vi "Open LVM Data.vi"(0 "Filename":path=path "E:/LabVIEW/Data/Test Data/Subj-Austin_Trial-1_Condition-None.lvm", 1 "VI reference":refnum<vi>, 11 "Error In":errorcluster) -> (4 "Filename Out":path=path "E:/LabVIEW/Data/Test Data/Subj-Austin_Trial-1_Condition-None.lvm" caption="Filename", 6 "All Data":dynamicdata(graph), 10 "EGG?":bool, 15 "Error Out":errorcluster)   [LabVIEW 2020]
panel:
  out "Signals (Array)":string[](array[string])
  out "EGG":dynamicdata(graph)
  out "Upper SPL":dbl
  out "Comment":string
  out "Audio":dynamicdata(graph)
  out "SPL":dynamicdata(graph)
  out "Pressure":dynamicdata(graph)
  out "Flow":dynamicdata(graph)
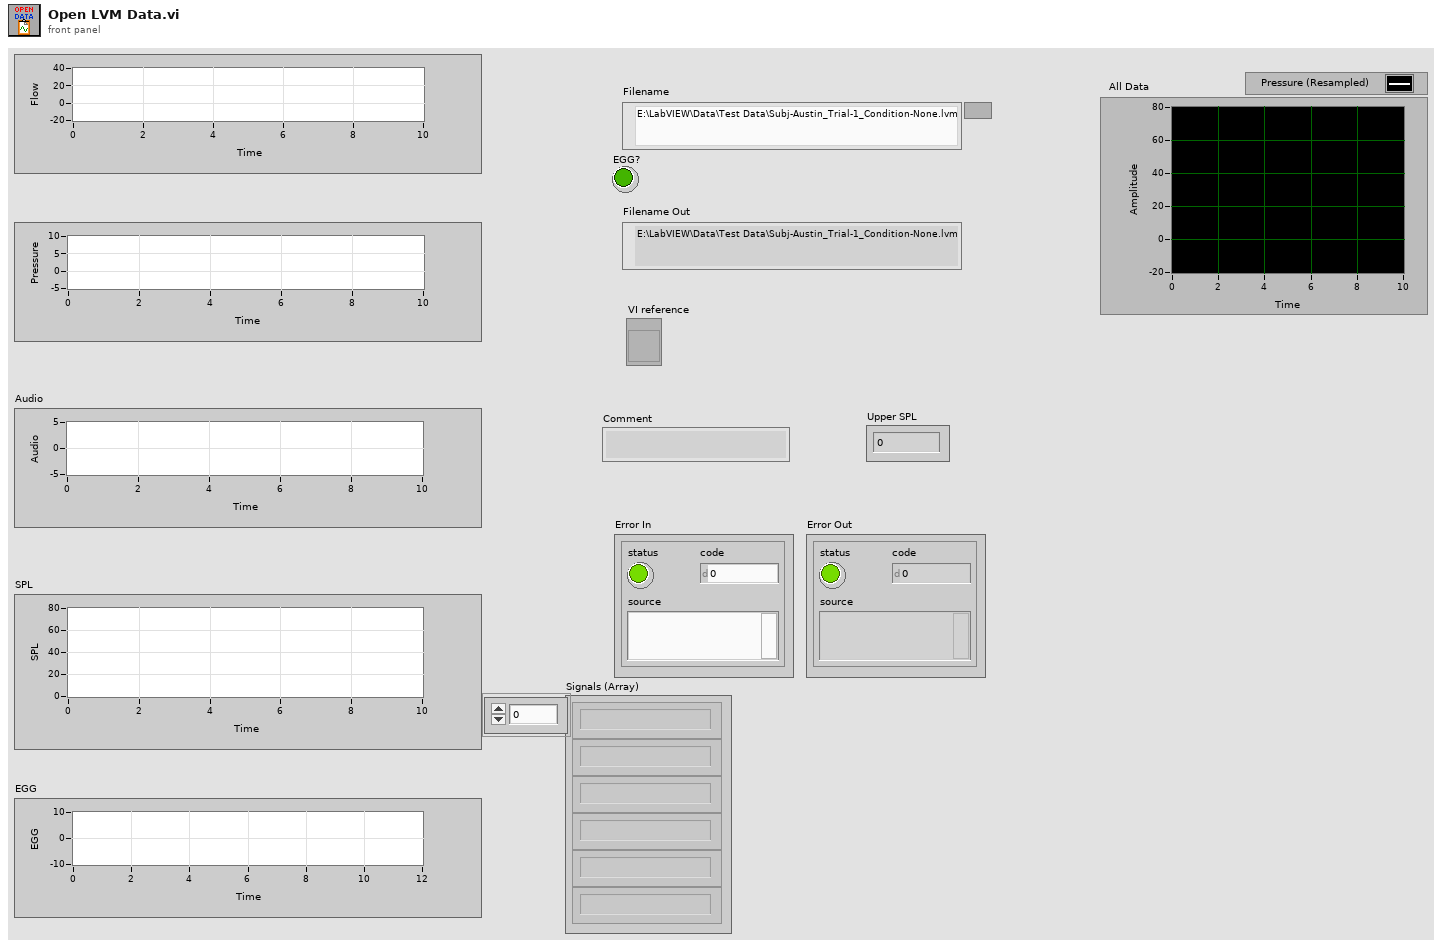
[diagram p1: front panel]
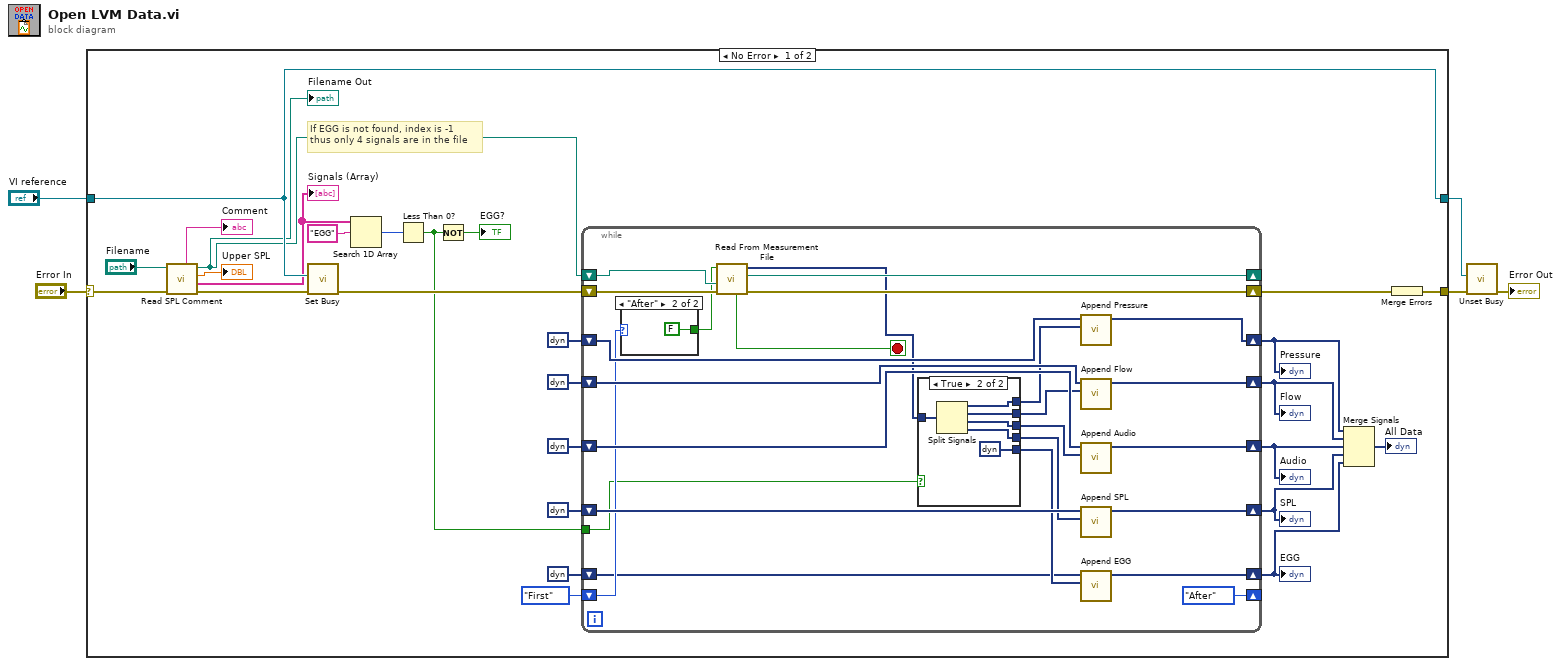
[diagram p0: block diagram]
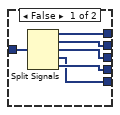
[diagram p2: hidden frame]
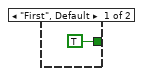
[diagram p3: hidden frame]
diagram:
  n1 = case shown="No Error" "Error In" {
    selector: "Error In" -> [w20 w73]
    tunnel: [w32 w73] -> w4
    tunnel: "VI reference" -> [w25 w72]
    tunnel: [w25 w72] -> w1
    frame No Error {
      # "If EGG is not found, index is -1\nthus only 4 signals are in the file"
      n2 = call "Read SPL Comment.vi"("error in (no error)"=w20, "Filename"="Filename") -> ("error out"=w14:errorcluster, "Signals"=w15:string[], "Upper SPL"=→"Upper SPL":dbl, "Filename Out"=w17:path, "Comment"=→"Comment":string)  [unwired: 5 in]
      "Filename Out" <- w17
      "Signals (Array)" <- w15
      n3 = call <vilib>:"Set Busy.vi"("error in (no error)"=w14, "VI reference (current VI)"=w25) -> ("error out"=w21:errorcluster)  [unwired: 8 in, 1 out]
      n4 = Search 1D Array(1D array=w15, element="EGG") -> (index of element=w22:i32)  [unwired: 1 in]
      n5 = Less Than 0?(x=w22) -> (x < 0?=w13:bool)
      n6 = Not(x=w13) -> (.not. x?=→"EGG?":bool)
      n7 = while {
        shift-right: [w56] -> w27
        shift-left: w21 -> [w55]
        shift-right: [w57] -> _
        shift-left: w17 -> [w54]
        shift-right: [w45] -> w11
        shift-left: dynamicdata [] ("Waveform Graph") -> [w52]
        shift-right: [w41] -> w10
        shift-left: dynamicdata [] ("Waveform Graph") -> [w51]
        shift-right: [w44] -> w9
        shift-left: dynamicdata [] ("Waveform Graph") -> [w50]
        shift-right: [w42] -> w8
        shift-left: dynamicdata [] ("Waveform Graph") -> [w49]
        shift-right: [enum16{"First", "After"}."After"] -> _
        shift-left: enum16{"First", "After"}."First" -> [w40]
        shift-right: [w34] -> w7
        shift-left: dynamicdata [] ("Waveform Graph") -> [w35]
        tunnel: w13 -> [w33]
        stop <- w53 stop-if-true
        n8 = case shown="\"After\"" w40 {
          tunnel: [TRUE ("Reset") FALSE ("Reset")] -> w39
          frame "First", Default {
          }
          frame "After" {
          }
        }
        n9 = call "Read From Measurement File"("error in (no error)"=w55, "Filename"=w54, "Reset"=w39) -> ("error out"=w56:errorcluster, "Filename Out"=w57:path, "Signals"=w43:dynamicdata, "EOF?"=w53:bool)  [unwired: 3 in, 2 out]
        n10 = case shown="True" w33 {
          tunnel: [w63 w67] -> w48
          tunnel: [w62 w66] -> w47
          tunnel: [w61 w65] -> w46
          tunnel: w43 -> [w60 w69]
          tunnel: [w59 w64] -> w37
          tunnel: [w58 dynamicdata [] ("Waveform Graph")] -> w36
          frame False {
            n11 = Split Signals(w60) -> (w63:dynamicdata, w62:dynamicdata, w61:dynamicdata, w58:dynamicdata, w59:dynamicdata)  [unwired: 5 in]
          }
          frame True {
            n12 = Split Signals(w69) -> (w67:dynamicdata, w66:dynamicdata, w65:dynamicdata, w64:dynamicdata)  [unwired: 4 in]
          }
        }
        n13 = call "Append Pressure"("Input Signal B"=w48, "Input Signal A"=w52) -> ("Appended Signals"=w45:dynamicdata)  [unwired: 8 in, 1 out]
        n14 = call "Append Flow"("Input Signal B"=w47, "Input Signal A"=w51) -> ("Appended Signals"=w41:dynamicdata)  [unwired: 8 in, 1 out]
        n15 = call "Append Audio"("Input Signal B"=w46, "Input Signal A"=w50) -> ("Appended Signals"=w44:dynamicdata)  [unwired: 8 in, 1 out]
        n16 = call "Append SPL"("Input Signal B"=w37, "Input Signal A"=w49) -> ("Appended Signals"=w42:dynamicdata)  [unwired: 8 in, 1 out]
        n17 = call "Append EGG"("Input Signal B"=w36, "Input Signal A"=w35) -> ("Appended Signals"=w34:dynamicdata)  [unwired: 8 in, 1 out]
      }
      "Flow" <- w10
      "Pressure" <- w11
      "SPL" <- w8
      "Audio" <- w9
      "EGG" <- w7
      n18 = Merge Signals(w11, w10, w9, w8, w7) -> (→"All Data":dynamicdata)
      n19 = Merge Errors(w27) -> (w32:errorcluster)
    }
    frame Error {
    }
  }
  n20 = call <vilib>:"Unset Busy.vi"("error in (no error)"=w4, "VI reference (current VI)"=w1) -> ("error out"=→"Error Out":errorcluster)  [unwired: 9 in]
